vi "ObtainPrivateQueues.vi"(8 "error in (no error)":errorcluster, 11 "Generator":refnum<class "Generator.lvclass">) -> (0 "error out":errorcluster, 3 "Generator out":refnum<class "Generator.lvclass">)   [LabVIEW 2019, in "Generator.lvclass"]
uses:
  Generator.lvclass
  Generator.lvclass/Generator.ctl
  typedefs/Message--Cluster.ctl
panel:
  # "For instructions on how to use the JKI State Machine Objects, examples and video tutorials, visit:\nhttp://jki.net/state-machine-objects/\n\nJKI State Machine Objects™\nhttp://jki.net/state-machine-objects/\nCopyright (C) 2005-2015, JKI <info@jki.net>\nALL RIGHTS RESERVED"
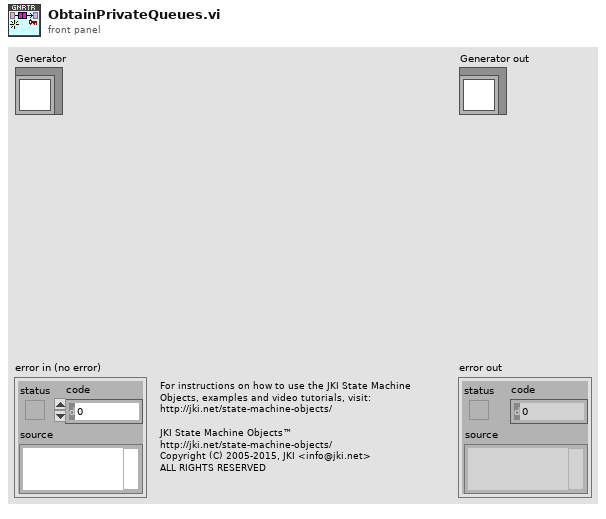
[diagram p1: front panel]
types:
  T1 = typedef "Generator.lvclass/Message--Cluster.ctl" = cluster{"Command":string, "Data":variant}
  T2 = typedef "Generator.lvclass/AO.Channel--Cluster--Array.ctl" = T3[]
  T3 = typedef "Generator.lvclass/AO.Channel--Cluster.ctl" = cluster{"Enable?":bool, "Channel":i32, "Amplitude":dbl, "Offset":dbl, "Frequency":dbl, "Phase":dbl, "Function":T4, "Sweeping?":bool, "Limit AC":bool, "Limit DC?":bool}
  T4 = typedef "Generator.lvclass/AO.Channel.Function--Enum.ctl" = enum16{"Sine", "Triangle", "Square"}
  T5 = cluster{"Enable?":bool, "Channel":i32, "Frequency":dbl, "Phase":dbl, "TC":dbl, "Roll-Off":i32}[]
  T6 = typedef "Generator.lvclass/Sweep.Configuration--Cluster.ctl" = cluster{"Sweep Time (s)":dbl, "Initial Wait (s)":dbl, "Return to Start":bool, "Channels":T7}
  T7 = typedef "Generator.lvclass/Sweep.Channel--Cluster--Array.ctl" = T8[]
  T8 = typedef "Generator.lvclass/Sweep.Channel--Cluster.ctl" = cluster{"Enable?":bool, "Channel":u16, "Start":dbl, "End":dbl, "Pattern":T9, "Table":dbl[]}
  T9 = typedef "Generator.lvclass/Sweep.Pattern--Enum.ctl" = enum16{"Ramp /", "Ramp /\\", "Smooth Ramp _/", "Smooth Ramp _/\\_", "Table"}
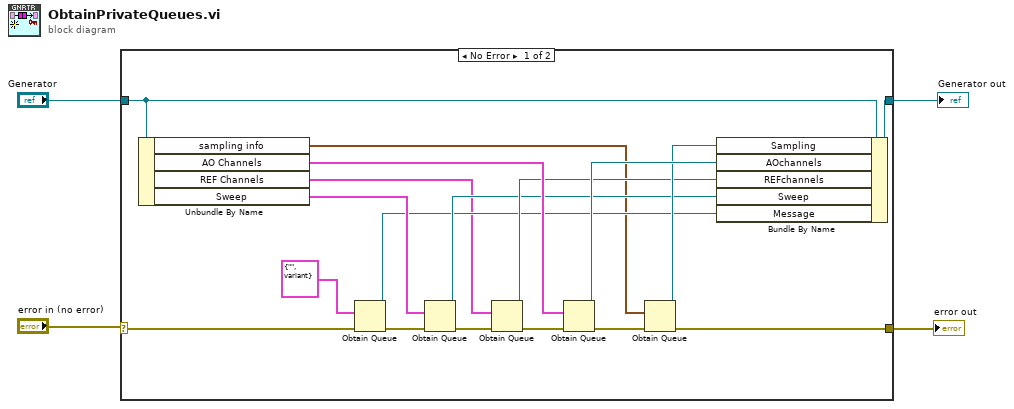
[diagram p0: block diagram]
diagram:
  n1 = case shown="No Error" "error in (no error)" {
    selector: "error in (no error)" -> [w13 w24]
    tunnel: [w12 w24] -> w2
    tunnel: [w22 w23] -> w3
    tunnel: "Generator" -> [w21 w23]
    frame No Error {
      n2 = Unbundle By Name(w21) -> ("sampling info"=w6:cluster{"Fs":dbl, "#s":dbl}, "AO Channels"=w18:T2, "REF Channels"=w5:T5, "Sweep"=w19:T6)
      n3 = Obtain Queue(element data type=T1 {"Command"="", "Data"=variant} ("Message"), error in (no error)=w13) -> (queue out=w7:refnum<queue>, error out=w17:errorcluster)  [unwired: 3 in, 1 out]
      n4 = Obtain Queue(element data type=w19, error in (no error)=w17) -> (queue out=w8:refnum<queue>, error out=w16:errorcluster)  [unwired: 3 in, 1 out]
      n5 = Obtain Queue(element data type=w5, error in (no error)=w16) -> (queue out=w9:refnum<queue>, error out=w15:errorcluster)  [unwired: 3 in, 1 out]
      n6 = Obtain Queue(element data type=w18, error in (no error)=w15) -> (queue out=w11:refnum<queue>, error out=w14:errorcluster)  [unwired: 3 in, 1 out]
      n7 = Obtain Queue(element data type=w6, error in (no error)=w14) -> (queue out=w10:refnum<queue>, error out=w12:errorcluster)  [unwired: 3 in, 1 out]
      n8 = Bundle By Name(cluster=w21, "Sampling"=w10, "AOchannels"=w11, "REFchannels"=w9, "Sweep"=w8, "Message"=w7) -> (w22:refnum<class "Generator.lvclass">)
    }
    frame Error {
    }
  }
  "error out" <- w2
  "Generator out" <- w3
